vi "Parse.vi"(8 "Error In":errorcluster, 11 "object in":refnum<class "2021_4.lvclass">) -> (0 "Error Out":errorcluster, 3 "object out":refnum<class "2021_4.lvclass">)   [LabVIEW 2020, in "2021_4.lvclass"]
uses:
  2021_4.lvclass
  2021_4.lvclass/2021_4.ctl
panel:
  out "min value":u32
  out "max value":u32
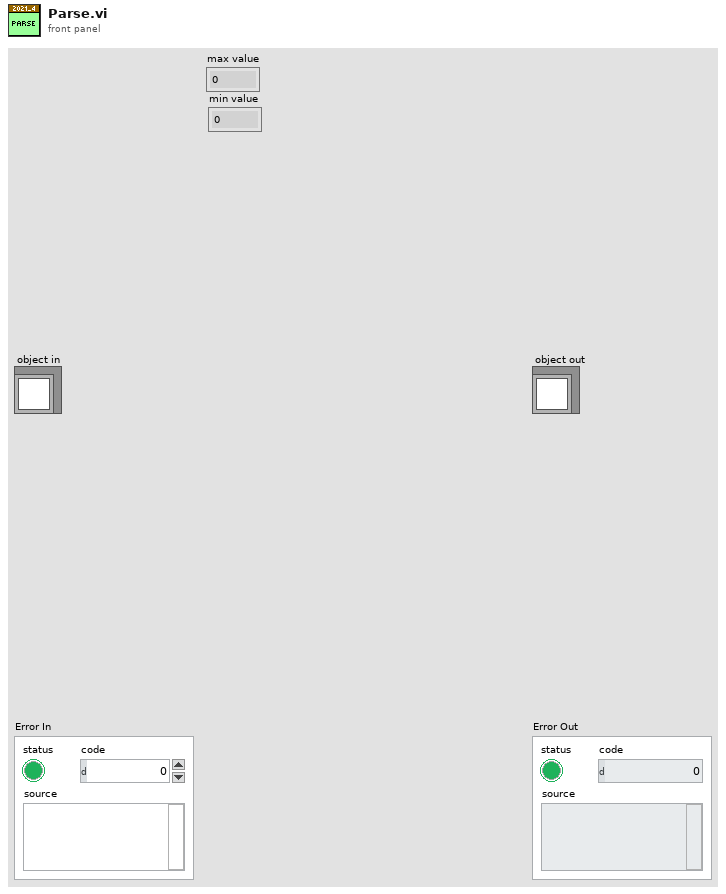
[diagram p1: front panel]
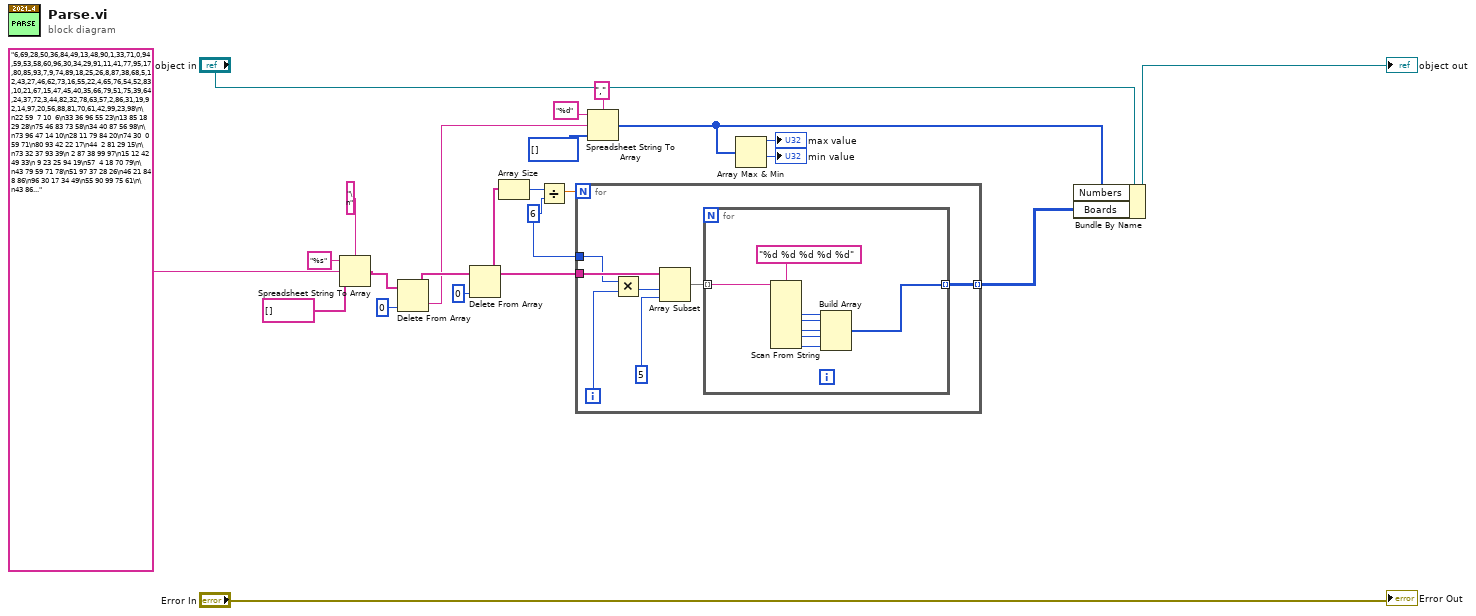
[diagram p0: block diagram]
diagram:
  w9 = 6 ("y")
  n1 = Spreadsheet String To Array(delimiter (Tab)="\n", format string="%s", spreadsheet string="6,69,28,50,36,84,49,13,48,90,1,33,71,0,94,59,53,58,60,96,30,34,29,91,11,41,77,95,17,80,85,93,7,9,74,89,18,25,26,8,87,38,68,5,12,43,27,46,62,73,16,55,22,4,65,76,54,52,83,10,21,67,15,47,45,40,35,66,79,51,75,39,64,24,37,72,3,44,82,32,78,63,57,2,86,31,19,92,14,97,20,56,88,81,70,61,42,99,23,98\n\n22 59  7 10  6\n33 36 96 55 23\n13 85 18 29 28\n75 46 83 73 58\n34 40 87 56 98\n\n73 96 47 14 10\n28 11 79 84 20\n74 30  0 59 71\n80 93 42 22 17\n44  2 81 29 15\n\n73 32 37 93 39\n 2 87 38 99 97\n15 12 42 49 33\n 9 23 25 94 19\n57  4 18 70 79\n\n43 79 59 71 78\n51 97 37 28 26\n46 21 84  8 86\n96 30 17 34 49\n55 90 99 75 61\n\n43 86 35 51 24\n16 25 29 21  3\n 2 13  4 36 54\n89 27  8 85 34\n96 59 65 14 56\n\n 5 57 43  4  1\n86 80 67 30 20\n22 16 99  0 14\n40 25 59 91 54\n82 95 96 37 24\n\n97 20 87 66 21\n25 40  9 78 89\n52 75 95 63 62\n32 43 13 47 69\n53 48 56 29  4\n\n24  4 65 12  8\n76  3 81 99 49\n45 33 31 66 34\n17 94 75 35 88\n64 10  7 93 95\n\n88 20 99 15 83\n81 40  5  6 98\n49 74 18 27  9\n43 69 28 37 71\n87 82 90 14 47\n\n21 97 92 42 60\n11 65 98 95 29\n 2 49 75 20 74\n56 40 78 66 81\n68  4 46 77 61\n\n26 14 39 76 11\n41 74 34 91  4\n51  9 97 29 75\n83 86 23 35 77\n90  2 49 30 89\n\n34 97  0 22 15\n65 60 82 66 47\n30  9 49 95 48\n54 73 67 17 78\n33 96 44  1 32\n\n90 29 10 49 63\n 8 26 95 61  0\n54 13 51 12 44\n32 48 16 47 84\n55 46 93 14  3\n\n68 55 46 16 54\n97 59 49  6 21\n52 32 15 96 70\n57 56 61 51  0\n40 31 62 24 48\n\n75 56 70 42 14\n77  9 23 62 25\n29 27 54 17  2\n55 72 43 15 96\n45 30 88 86  1\n\n65 12 22  6 51\n77 81 15 91 19\n80 71 27 89 52\n75 92 41 83 57\n40 44 66 84 98\n\n89 80 73 59 18\n74 55 67 71 10\n78 27 37 57  3\n92 26 17  5 72\n52 83 28 76 51\n\n64  0 87  4 13\n14 43 42 62 31\n17 84 72 91 83\n53 80 59 61 74\n47 22 38 28 77\n\n65 49 91 94 19\n25 81 64 57  9\n50 95 82 12 66\n53 54 85 36 11\n31 56 83 18 60\n\n 6 12 76 37 33\n14 96 16 31 40\n17 82 27 94 83\n 1 50 49  9 54\n29 70 59 91 77\n\n85  0 33 41 16\n 7 86 80 53 65\n94 19 28 35 32\n 4 55 93 97 63\n83 22 67 56 36\n\n28 70 65 17 19\n88 51 15 73 12\n11 49 80 23 42\n26 54 90 75 29\n74 77 91 86 66\n\n88 22 83 10 43\n57 34 15 23  8\n94 42 68 67 37\n84  3  6 71 62\n89 45 72 55 38\n\n68 27 93  7 15\n85 96  1 56  6\n32  2 30 55 17\n99 90 37 80 50\n77 78 58 98 57\n\n 5 95 22 13 97\n19  2 52 92 20\n75 49 86 31 41\n51 63 56 33 10\n82 27 79 94 57\n\n15 44 91 26  4\n41 78 53 95 86\n90 92 46 56 33\n80 93 68 66 70\n36 10 38  0  6\n\n11 47 52 64 17\n16 60 39 55 78\n46 18 33 83 35\n13 92  4 23 50\n40  5 29  6 90\n\n20 60  2 23 74\n43 39 91 75 12\n58 67 50 29 79\n10 40 92 95 25\n13 24 53 72 36\n\n69 64 15 53 86\n61 11 48 71 27\n26 93 38 70 73\n96 29 30 98 45\n13  7 31 59 84\n\n13 55 50 54 57\n32 24 45  5 77\n82 86  0  4 99\n75 72 14 40 56\n76 94 89 17 30\n\n66 71 86 41  0\n80 64  3 29 78\n23 21 42 99 87\n96 60 75 61 49\n 2 83 85 12  1\n\n78 96  4 82  6\n73 36 57 99  8\n11 83 15 35 30\n85 87 25 22 66\n32 64 16 50 43\n\n 6 39 55  2  4\n 1 61 99 71 80\n46 88 22 31 60\n62 66 37 97 76\n74 34 10 52 24\n\n42 38 13 65 12\n 4 39 60 62 21\n81 99  1 69 40\n59 15 11 95 53\n91 78 72 30 73\n\n43 68 82 72  2\n34 92 33 97 89\n63 70  9  0 45\n69 10 12 65 21\n40 20 55 57 49\n\n41 22  8 16 49\n71 64 19 65 92\n17 10 26 36 29\n30 88  7 54 11\n77 55 70 72 47\n\n15 94 90  6 39\n99 55 16 54 91\n18  7 82 44 51\n25 34 83 14 12\n30  2 77 27 66\n\n44 50 74 97 58\n87 42 56 92 28\n49 82 52 17 78\n54 89 63 77 27\n83 14 24 16 84\n\n47 32  8 55 22\n19 14 24 82  4\n76 73  9 10 64\n40  6 92 67 17\n68 44 43  3 54\n\n26 10  9 92 81\n46 98 13  0 14\n68 99 35 18 72\n74 33 22 61 93\n80 38 71  6 75\n\n17 23 54 55 22\n10  8 60 76 24\n71 28 16 62 82\n13 12 21 78 39\n26 66 89 64 79\n\n72 12 91 79 99\n84 18 37 98 41\n10 71 88 23 24\n11 34 26 83 74\n58 27 77  5  8\n\n 9 90 13  0 46\n 6 58 74 92  8\n75 77 56 76 80\n55 60 44 68 91\n67 28 96 66 18\n\n14 26 54 21 35\n69 67 16 76 62\n78 45 87 44 94\n27 89 39 85 28\n 3 81 93 64 74\n\n10 28 35 84 76\n40 11 95 59 57\n53  4 24 50 45\n 7 43 78 17 81\n 1 74 82 16 27\n\n 6 26 72 53 52\n51 91 80 11 18\n20 63 74 25 33\n79  4  8 59 67\n 3 13 55 81 83\n\n98 85 27 84 42\n90 15 17 61 34\n40 64 86 96 45\n59 47 53  5 35\n11  7 41 80 13\n\n47 48 54 31 76\n99 32 98 20 15\n61 41 30 94 37\n34 59 86 55 45\n 9 83 92 53  3\n\n 3 80 24 94 25\n17 23 64 76 71\n20 97  0 56 72\n95 73 28 59 21\n14 81 46 67 88\n\n 2 95  5 38 90\n63 62 11 24 34\n19 31 57 84 80\n47 86 36 85 74\n13 39 73 94 42\n\n28  6 60 34 15\n63 36 51 30 92\n43 10  7 88 49\n78 76 31 19 66\n22 20 35 45 79\n\n19 42 49 57 73\n99 50 97 93 43\n67 52 40 16 33\n 2 55  0 71 46\n21 75 59 66 83\n\n19 86 30 25  3\n32 39 65 54 29\n38  6 85 52 13\n43 95 18 44 15\n53 70 16 31 71\n\n68 73 74 83 70\n56 15 12 78  4\n43 87 63 90 86\n41 16 23 17 77\n80 14 61 30 50\n\n88 28 45 80 65\n64 11 68 33 27\n29 70 44 82 37\n42 66  9 32 87\n10 24 15  3 46\n\n99 81  5 62 97\n 4 36 23 38 35\n42 16 37 98 54\n34 41 25 30 48\n 8 60 63 89 72\n\n25 33 94 23 14\n45 10 79 30  3\n22 28 95 27 11\n74 13 39 84 83\n72 88 56 53 97\n\n31 92 91 84 71\n54 90 89 80  0\n98 96 65 66 68\n35 39 70 11 82\n15 34 42 52  2\n\n68 71 86 82 37\n28 48 12 34 54\n62 55 10 25 89\n60  4 50 21 22\n 3  2 18 40 84\n\n18 96 95 47 45\n14 51  2 88 43\n94 56 19 15  8\n48 65 62  6 75\n35 28 25 72 30\n\n43 85 69 92 26\n61 75  5 73 66\n16 87  4 99 48\n18 19 79 23 83\n37 88 31 38 40\n\n23 10 89 84 76\n45 39 62 55 66\n25 73 79 43 60\n12 69 36 93 71\n 9 77 14 58 49\n\n 9 24 26 53 79\n99 15 30 50 16\n14 95 12 25 33\n54 40 58 46 66\n 5 23 39 29 48\n\n64 67 11 10 92\n59 99 80 97 66\n45 51 88 47 82\n35 27 72 85 16\n54 58  2  1 52\n\n10 97 27 54 66\n89 85 39 99 98\n 8 68 95 51 19\n 4 17 79 87  3\n72 43 76 58 33\n\n95 72  0 18 17\n 3 42 24 86 34\n52 79 46 58 98\n76 77 78 19 10\n81 61 88 85 54\n\n74 70 15 80 72\n77 89 11 19 22\n34 59 56 65 91\n58  6 50 40 16\n93 30 95 26 85\n\n47 62 57  6 25\n40 79 22 95 29\n42 11 70 10 92\n60 53 84 96 17\n75 86 74 89 18\n\n30 42  4 19 92\n40 58 72  7 70\n17 98 45 76 50\n93 57 65 79  2\n56 94 73 84 62\n\n51  0 14  7 53\n63 36 48 81 84\n50 22 11 88  6\n83 99 21 31 91\n86 17 72 42 94\n\n83  0 20 26  7\n42 24 37 86 65\n73 82 63 21 27\n30 35  9 47 80\n79 53  3 14 84\n\n50 99 83 86 42\n81 36 24  4 76\n 0 71 66 41 57\n 7 54 94 78 97\n12  8 82 45 31\n\n 4 91 57 50 37\n22 46 86 24 26\n39 54 48  7 42\n 2 45 95 29 12\n38 25 52  0 72\n\n51 94 46 44 62\n95 60  0 48 61\n38 13 85 32  8\n22 56 53 30 80\n43 65 58 68 88\n\n49 76 41 43 51\n57 46 45 82 90\n48 33 36  5 23\n81 30  3 61 75\n56 70 29 91 59\n\n58 74 50 47 84\n 2  1 62 36 60\n32 16 95 43 27\n79 12 39 56 11\n 9 33  4 25 61\n\n23 84 16 51 39\n72 19 53 64 43\n 9 44 10 52 26\n45 68 29 56 74\n62 42 46 95  0\n\n16 83 27 85 56\n13 41 49 79 53\n18 63  7 60  3\n45 15 48 69 29\n46 86 35 34 32\n\n85  2 96 15 43\n33 30 29 53 98\n21 55 61 73 40\n31  4 66 75 59\n26 32 91 38 80\n\n69 81 65 30 77\n82 22 83  0 38\n 2  3 29 47 94\n42 55  9 18 97\n53 45 90 31 44\n\n23 86  0 35 84\n27 80  3 64 12\n 1 96 48 93 85\n69 24 61 15 22\n91 72 62 13 76\n\n81 51 67 60 16\n65 48 86 39 97\n92 93 49 77 59\n15 94 88 52 19\n80 83 23 61  4\n\n47 84 46 79 55\n92 38 65 42 76\n 9 58 26 95 86\n30 49 56 69 59\n94  4 25 89 44\n\n73 10 29  0 48\n56 40 19 84 61\n52 31 25 86 21\n79 55 53 51  5\n81  9 35 72 15\n\n41 95 30 58 73\n26 80  4 21 96\n61 92 76 93 74\n 2 69 60  8 20\n46 98 70 72 83\n\n 1 99 31  4 86\n93 64  8 43 61\n33 36 75 90 50\n52 13  3 42 34\n22 65 60 18 76\n\n17 63  6 66 92\n51 67 86 88 18\n82 83 32 74 30\n 5 33  9 28 61\n72 75 25 23 60\n\n43 28 40 53 52\n54 12 77 10 83\n21 44 63  0  1\n15 22 33 49  2\n80 41  3 46 55\n\n 1 97 75 37  4\n47 33 13 21 40\n27 62 15 90 30\n11 83 63 36 35\n 0 12 60 91 42\n\n 0 45 17 88 18\n66 10 63 62  8\n36  5 47 39 67\n21  3 61 29 19\n82 58 33  6 59\n\n37 92 69 56 52\n46 66 20 78 13\n83 99 16 31  0\n36 35  2 68  9\n70 82 94 96 29\n\n62 65 85 37  3\n74 95 34 96 58\n15 33 49 21 93\n19 83 66  6 25\n81 84 23  0 76\n\n95 84 71 92 52\n54 36 66 59 82\n 0 76 32 45 83\n69 27 25 88 38\n81 96 63  4 61\n\n73 51 28 48 40\n 3 38 11 14 35\n66 91 86 20 81\n53 39 46 71  1\n97 60 21 93 23\n\n92 70  4 60 95\n58 49 20 15 25\n55 68 21 84 80\n56 41 82 23 19\n30 74 65 27 29\n\n81 97 68 46 75\n62 73 63 36 41\n 1  5 91 84 37\n45 92 20 49  7\n25 26  3 88 56\n\n25  9 94 37 26\n44 58 84 91 38\n39 46 57 98 50\n96 42 73 24 70\n71 32 53 48 13\n\n98 72 25 96 77\n80 64 88 53 23\n21 37 45 24 18\n41 86 59 68  5\n76 50 36 26 12\n\n77 79 88 74 12\n21  9 85 26 68\n11 62 64  4  5\n47 33 76 63 87\n55 19  2 60 95\n\n74 79 30 14 35\n90 52 17 29 63\n18 69 78 34 26\n92 42 85 71 56\n12  2  5  0 98" ("PuzzleInput"), array type (2D Dbl)=string[] []) -> (array=w16:string[])
  n2 = Delete From Array(array=w16, index=0) -> (deleted portion=w6:string, array with subset deleted=w14:string[])  [unwired: 1 in]
  n3 = Delete From Array(array=w14, index=0) -> (array with subset deleted=w12:string[])  [unwired: 1 in, 1 out]
  n4 = Array Size(array=w12) -> (size(s)=w11:i32)
  n5 = Divide(x=w11, y=w9) -> (x/y=w10:dbl)
  n6 = for {
    N: w10 -> [_]
    tunnel: w12 -> [w30]
    tunnel: w9 -> [w27]
    tunnel: [w24] -> w4 mode=indexing
    i -> [w28]
    n7 = Multiply(x=w27, y=w28) -> (x*y=w29:i32)
    n8 = Array Subset(array=w30, index=w29, length=5 ("y")) -> (w25:string[])
    n9 = for {
      tunnel: w25 -> [w38] mode=indexing
      tunnel: [w31] -> w24 mode=indexing
      n10 = Scan From String(format string="%d %d %d %d %d", input string=w38) -> (output 1=w36:i32, output 2=w35:i32, output 3=w34:i32, output 4=w33:i32, output 5=w32:i32)  [unwired: 7 in, 3 out]
      n11 = Build Array(w36, w35, w34, w33, w32) -> (w31:i32[])
    }
  }
  n12 = Spreadsheet String To Array(delimiter (Tab)=",", format string="%d", spreadsheet string=w6, array type (2D Dbl)=u32[] []) -> (array=w3:u32[])
  n13 = Array Max & Min(array=w3) -> (max value=→"max value":u32, min value=→"min value":u32)  [unwired: 2 out]
  n14 = Bundle By Name(cluster="object in", "Numbers"=w3, "Boards"=w4) -> (→"object out":refnum<class "2021_4.lvclass">)
  "Error Out" <- "Error In"
